vi "3x3inBound.vi"(1 "jj":i32, 2 "ii":i32, 3 "j":i32, 4 "i":i32) -> (0 "inBound":bool)   [LabVIEW 2024]
uses:
  globalVar.vi
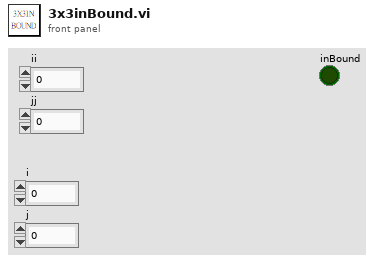
[diagram p1: front panel]
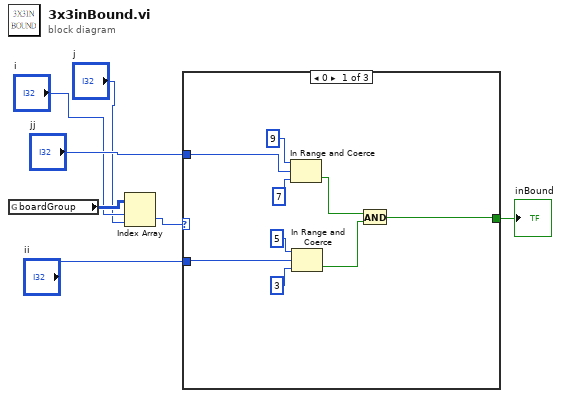
[diagram p0: block diagram]
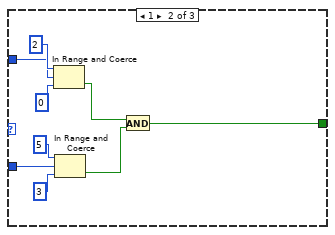
[diagram p2: hidden frame]
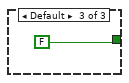
[diagram p3: hidden frame]
diagram:
  n1 = global read "globalVar.vi" "boardGroup"() -> (w7:i32[][])
  n2 = Index Array(array=w7, index (row)="i", index (col)="j") -> (element=w2:i32)
  n3 = case shown="0" w2 {
    tunnel: "ii" -> [w8 w19 _]
    tunnel: "jj" -> [w9 w18 _]
    tunnel: [w10 w17 FALSE] -> w1
    frame 0 {
      n4 = In Range and Coerce(upper limit=9, x=w9, lower limit=7) -> (In Range?=w15:bool)  [unwired: 1 out]
      n5 = In Range and Coerce(upper limit=5, x=w8, lower limit=3) -> (In Range?=w16:bool)  [unwired: 1 out]
      n6 = And(x=w15, y=w16) -> (x .and. y?=w10:bool)
    }
    frame 1 {
      n7 = In Range and Coerce(upper limit=2, x=w18, lower limit=0) -> (In Range?=w24:bool)  [unwired: 1 out]
      n8 = In Range and Coerce(upper limit=5, x=w19, lower limit=3) -> (In Range?=w25:bool)  [unwired: 1 out]
      n9 = And(x=w24, y=w25) -> (x .and. y?=w17:bool)
    }
    frame Default {
    }
  }
  "inBound" <- w1
